vi "Read State.vi"(11 "Stand in":refnum<class "Stand.lvclass">) -> (2 "State":T1)   [LabVIEW 2019]
uses:
  Stand.lvclass
  C:/Users/H4001/Documents/GitHub/H4000/src/Device_class/Device.lvclass
  C:/Users/H4001/Documents/GitHub/H4000/src/Proccess_class/Proccess.lvclass
  TypeDef/State.ctl
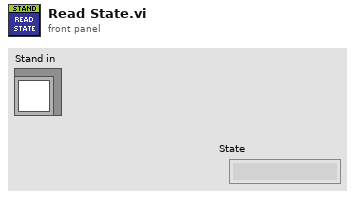
[diagram p1: front panel]
types:
  T1 = typedef "State.ctl" = enum16{""}
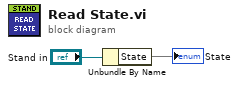
[diagram p0: block diagram]
diagram:
  n1 = Unbundle By Name("Stand in") -> ("State"=→"State")
